vi "ACal-Multiband Dialog.vi"(0 "Cluster In":T1 {"WF" items=["Chirp", "Noise"]}) -> (4 "Cluster out":T1 {"WF" items=["Chirp", "Noise"]}, 8 "Canceled?":bool)   [LabVIEW 2020]
uses:
  Type Defs/ACal-Multiband Parameters.ctl
panel:
  in  "WF":u16(ring) items=["Chirp", "Noise"]
  in  "Listbox":i32(listbox)
  in  "Max range (dB)":dbl
  in  "Fmax (Hz)":dbl
  in  "Fmin (Hz)":dbl
  out "Mag":cluster{"PTC Mag":dbl[], "PTC Phase":dbl[]}[](graph)
  in  "Folder":path
  in  "Cancel":bool
  in  "OK":bool
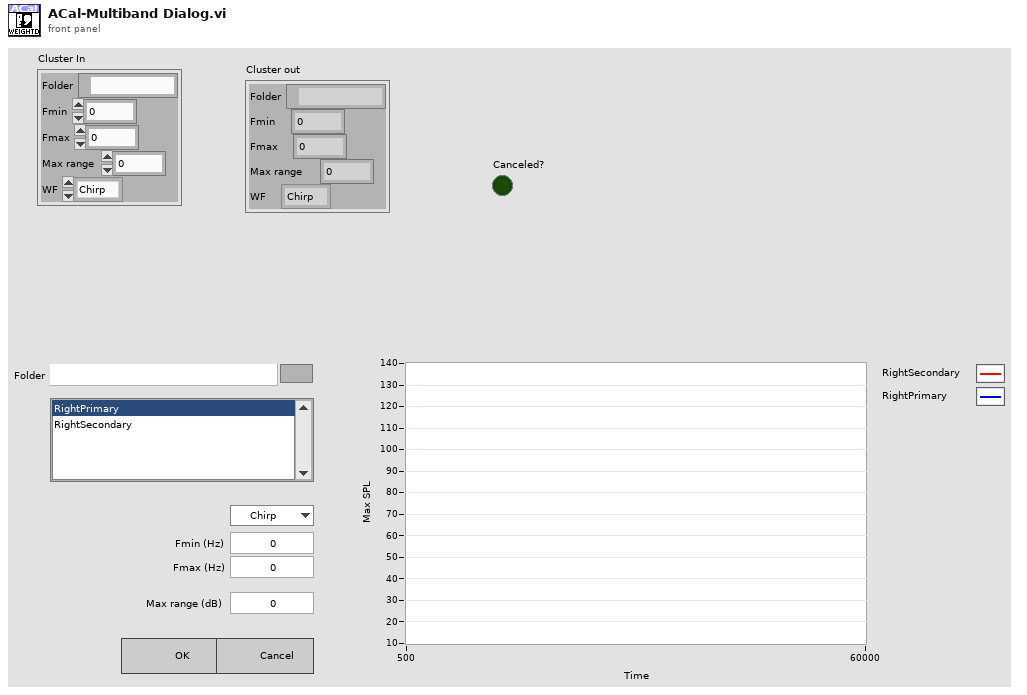
[diagram p1: front panel]
types:
  T1 = typedef "ACal-Multiband Parameters.ctl" = cluster{"Folder":path, "Fmin":dbl, "Fmax":dbl, "Max range":dbl, "WF":u16}
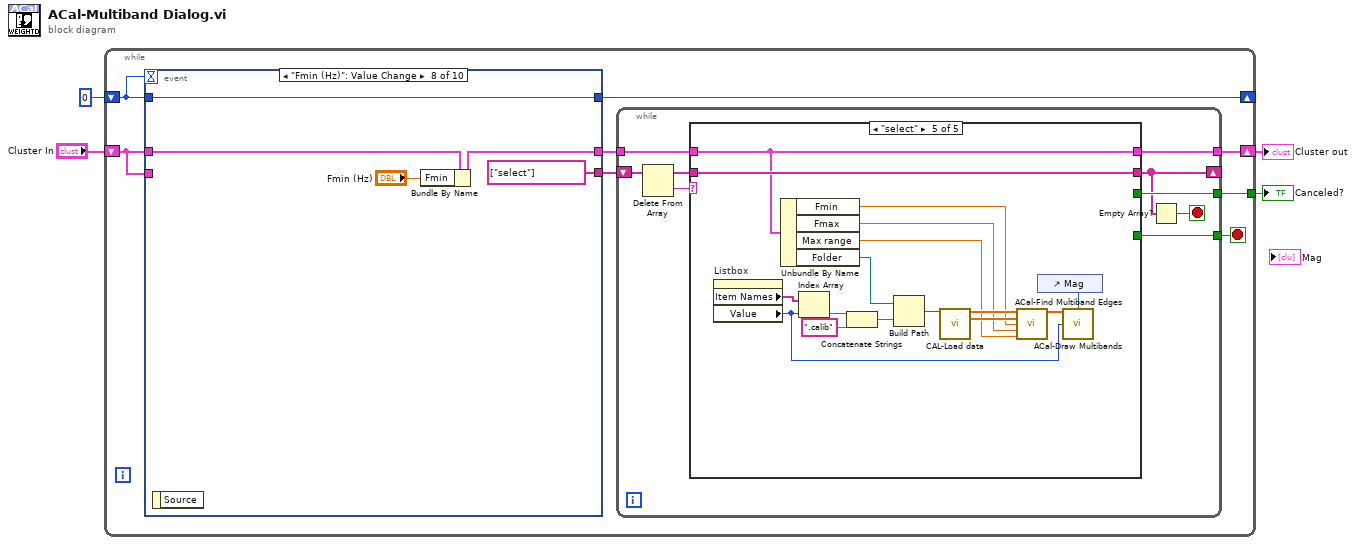
[diagram p0: block diagram]
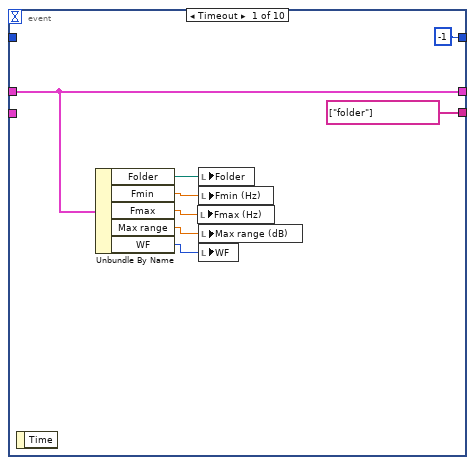
[diagram p2: hidden frame]
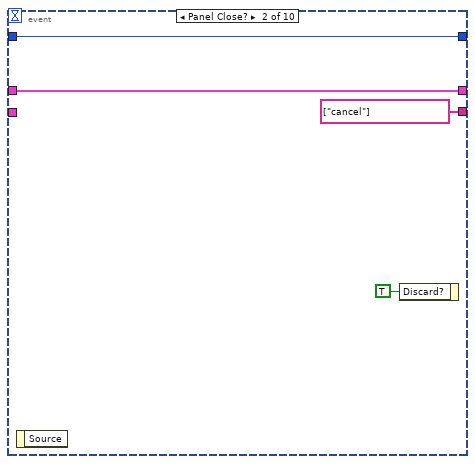
[diagram p3: hidden frame]
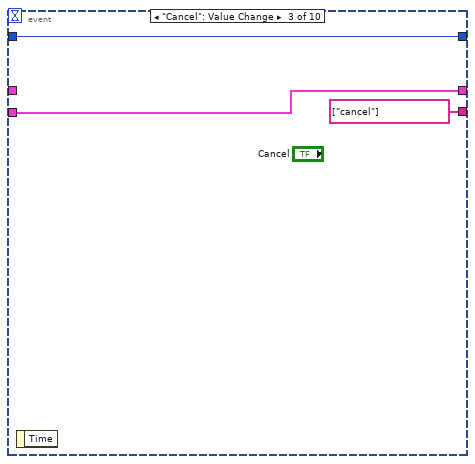
[diagram p4: hidden frame]
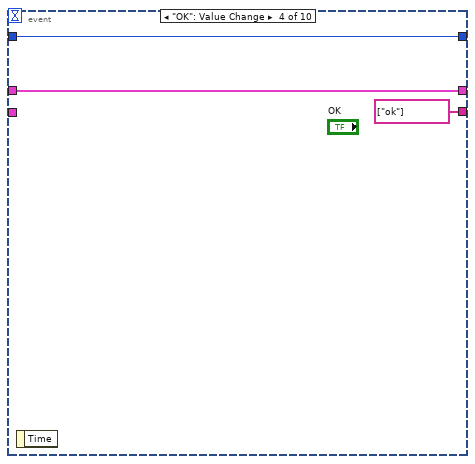
[diagram p5: hidden frame]
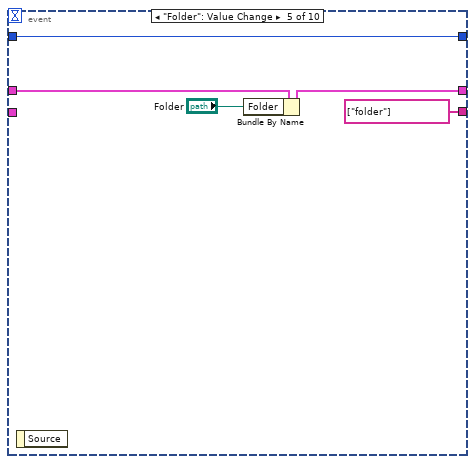
[diagram p6: hidden frame]
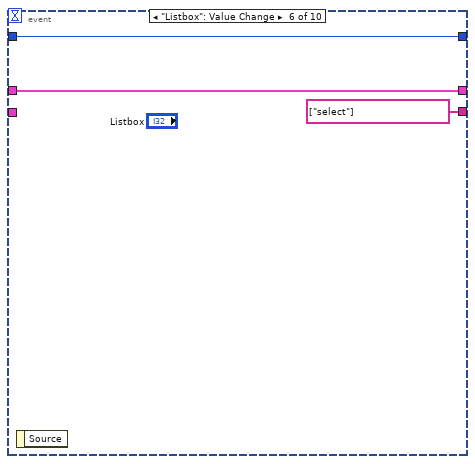
[diagram p7: hidden frame]
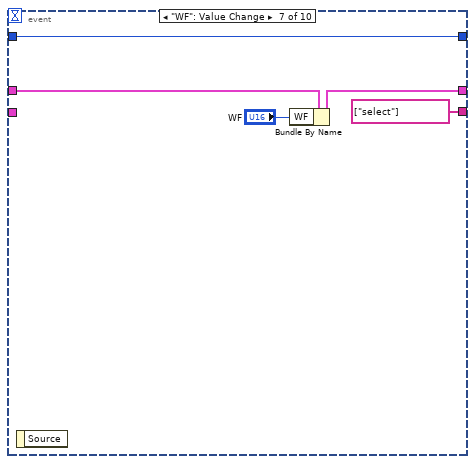
[diagram p8: hidden frame]
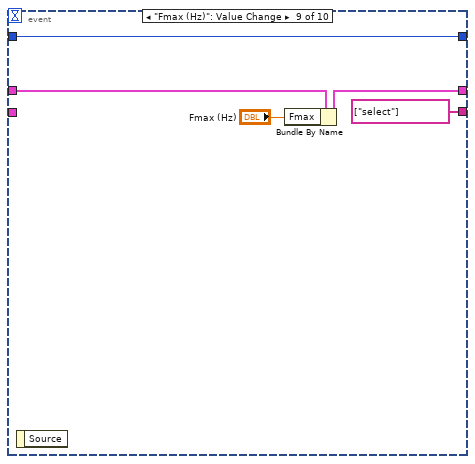
[diagram p9: hidden frame]
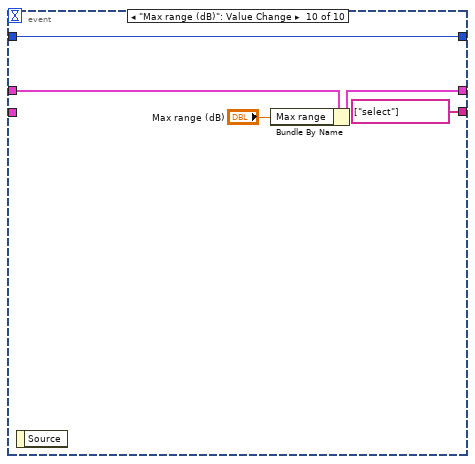
[diagram p10: hidden frame]
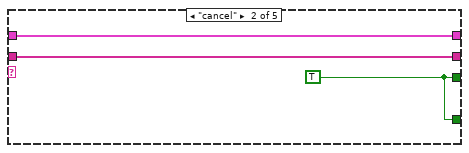
[diagram p12: hidden frame]
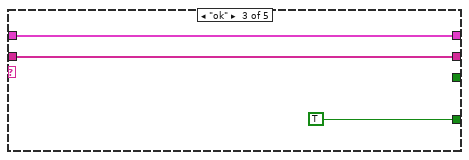
[diagram p13: hidden frame]
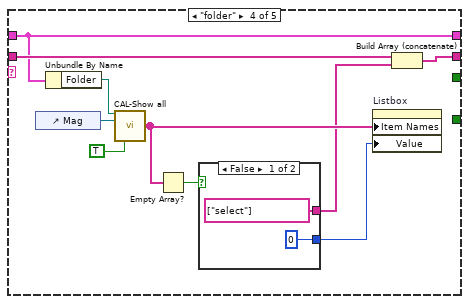
[diagram p14: hidden frame]
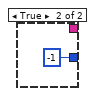
[diagram p15: hidden frame]
diagram:
  n1 = while {
    shift-right: [w12] -> _
    shift-left: 0 -> [w10]
    tunnel: [w6] -> w1
    shift-right: [w8] -> w2
    shift-left: "Cluster In" -> [w11]
    stop <- w5 stop-if-true
    n2 = event shown="[7] \"Fmin (Hz)\": Value Change" {
      selector: _ -> [_ _ _ _ _ _ _ _ _ _]
      dyn-events: _ -> [_ _ _ _ _ _ _ _ _ _]
      timeout: w10 -> [_ _ _ _ _ _ _ _ _ _]
      tunnel: [-1 w24 w26 w29 w35 w38 w43 w48 w53 w58] -> w12
      tunnel: w11 -> [w18 w23 _ w30 w34 w37 w42 w47 w52 w57]
      tunnel: [w18 w23 w27 w30 w33 w37 w41 w46 w51 w56] -> w9
      tunnel: w11 -> [_ _ w27 _ _ _ _ _ _ _]
      tunnel: w10 -> [_ w24 w26 w29 w35 w38 w43 w48 w53 w58]
      tunnel: [string[] ["folder"] string[] ["cancel"] string[] ["cancel"] string[] ["ok"] string[] ["folder"] string[] ["select"] string[] ["select"] string[] ["select"] string[] ["select"] string[] ["select"]] -> w7
      event Timeout {
        n3 = event-data() -> ()  [unwired: 1 in, 1 out]
        n4 = Unbundle By Name(w18) -> ("Folder"=w17:path, "Fmin"=w16:dbl, "Fmax"=w15:dbl, "Max range"=w14:dbl, "WF"=w13:u16)
        n5 = local write "Fmax (Hz)"(w15) -> ()
        n6 = local write "Folder"(w17) -> ()
        n7 = local write "Fmin (Hz)"(w16) -> ()
        n8 = local write "Max range (dB)"(w14) -> ()
        n9 = local write "WF"(w13) -> ()
      }
      event Panel Close? {
        n10 = event-data() -> ()  [unwired: 1 in, 1 out]
        n11 = event-data("Discard?"=TRUE) -> ()  [unwired: 1 in, 1 out]
      }
      event "Cancel": Value Change {
        n12 = event-data() -> ()  [unwired: 1 in, 1 out]
      }
      event "OK": Value Change {
        n13 = event-data() -> ()  [unwired: 1 in, 1 out]
      }
      event "Folder": Value Change {
        n14 = event-data() -> ()  [unwired: 1 in, 1 out]
        n15 = Bundle By Name(cluster=w34, "Folder"="Folder") -> (w33:T1)
      }
      event "Listbox": Value Change {
        n16 = event-data() -> ()  [unwired: 1 in, 1 out]
      }
      event "WF": Value Change {
        n17 = event-data() -> ()  [unwired: 1 in, 1 out]
        n18 = Bundle By Name(cluster=w42, "WF"="WF") -> (w41:T1)
      }
      event "Fmin (Hz)": Value Change {
        n19 = event-data() -> ()  [unwired: 1 in, 1 out]
        n20 = Bundle By Name(cluster=w47, "Fmin"="Fmin (Hz)") -> (w46:T1)
      }
      event "Fmax (Hz)": Value Change {
        n21 = event-data() -> ()  [unwired: 1 in, 1 out]
        n22 = Bundle By Name(cluster=w52, "Fmax"="Fmax (Hz)") -> (w51:T1)
      }
      event "Max range (dB)": Value Change {
        n23 = event-data() -> ()  [unwired: 1 in, 1 out]
        n24 = Bundle By Name(cluster=w57, "Max range"="Max range (dB)") -> (w56:T1)
      }
    }
    n25 = while {
      tunnel: w9 -> [w67]
      tunnel: [w66] -> w8
      shift-right: [w61] -> _
      shift-left: w7 -> [w65]
      tunnel: [w62] -> w6
      tunnel: [w59] -> w5
      stop <- w60 stop-if-true
      n26 = Delete From Array(array=w65) -> (deleted portion=w63:string, array with subset deleted=w64:string[])  [unwired: 2 in]
      n27 = case shown="\"select\"" w63 {
        tunnel: w67 -> [w69 w72 w75 w83 w98]
        tunnel: [w69 w72 w75 w83 w98] -> w66
        tunnel: [w68 w71 w74 w78 w104] -> w61
        tunnel: w64 -> [w68 w71 w74 w85 w104]
        tunnel: [_ w70 _ _ _] -> w62
        tunnel: [_ w70 TRUE _ _] -> w59
        frame "", Default {
        }
        frame "cancel" {
          w70 = TRUE
        }
        frame "ok" {
        }
        frame "folder" {
          n28 = control-ref of="Mag"() -> (w84:refnum<vi>)
          n29 = Unbundle By Name(w83) -> ("Folder"=w82:path)
          n30 = call "CAL-Show all.vi"("Path"=w82, "Mag graph"=w84, "Plot Max SPL"=TRUE) -> ("speakers"=w80:string[])  [unwired: 11 in, 1 out]
          n31 = Empty Array?(array=w80) -> (empty?=w79:bool)
          n32 = case shown="False" w79 {
            tunnel: [string[] ["select"] _] -> w77
            tunnel: [0 -1] -> w76
            frame False {
            }
            frame True {
            }
          }
          n33 = property on="Listbox" class="LstBox (strict)"("Item Names"=w80, "Value"=w76) -> ()  [unwired: 2 in, 2 out]
          n34 = Build Array (concatenate)(w85, w77) -> (w78:string[])
        }
        frame "select" {
          n35 = property on="Listbox" class="LstBox (strict)"() -> ("Item Names"=w103:string[], "Value"=w89:i32)  [unwired: 2 in, 2 out]
          n36 = Unbundle By Name(w98) -> ("Fmin"=w94:dbl, "Fmax"=w93:dbl, "Max range"=w92:dbl, "Folder"=w97:path)
          n37 = Index Array(array=w103, index=w89) -> (element=w102:string)
          n38 = Concatenate Strings(w102, ".calib" ("string")) -> (w99:string)
          n39 = Build Path(base path=w97, name or relative path=w99) -> (appended path=w100:path)
          n40 = call "CAL-Load data.vi"("user path"=w100) -> ("Frequency (Hz)"=w96:dbl[], "Mag"=w95:dbl[])  [unwired: 7 in, 6 out]
          n41 = call "ACal-Find Multiband Edges.vi"("Freq"=w96, "Mag"=w95, "Fmin"=w94, "Fmax"=w93, "Max Range"=w92) -> ("Fstart"=w91:dbl[])  [unwired: 8 in, 2 out]
          n42 = control-ref of="Mag"() -> (w90:refnum<vi>)
          n43 = call "ACal-Draw Multibands.vi"("Fstart"=w91, "XYGraph in"=w90, "Plot"=w89) -> ()  [unwired: 13 in]
        }
      }
      n44 = Empty Array?(array=w61) -> (empty?=w60:bool)
    }
  }
  "Cluster out" <- w2
  "Canceled?" <- w1
